vi "New File&Save Test Info_SubVIs-某型振动实验台测试系统.vi"(6 "测试条件":T3, 7 "粉尘特性":T2, 8 "error in":errorcluster, 9 "Task Info.Accele Task":T1[](array[typedef]), 11 "Test Info":cluster{"Test Name":string, "Tester":string}) -> (0 "error out":errorcluster)   [LabVIEW 2011]
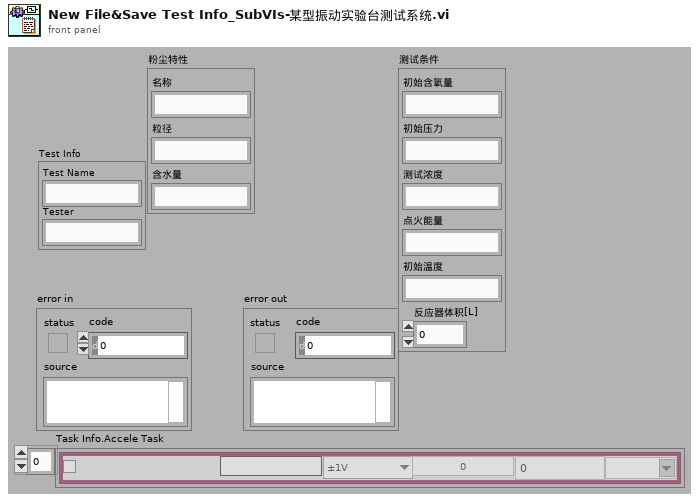
[diagram p1: front panel]
types:
  T1 = typedef "Acceleration Channel Config_Ctrls-某型振动实验台测试系统.ctl" = cluster{"Enable":bool, "Name":string, "range":enum16{"±1V", "±5V"}, "SensValue":dbl, "PhysicalName":string, "off":dbl, "Sensunits":string}
  T2 = typedef "粉尘特性.ctl" = cluster{"名称":string, "粒径":string, "含水量":string}
  T3 = typedef "测试条件.ctl" = cluster{"初始含氧量":string, "初始压力":string, "测试浓度":string, "点火能量":string, "初始温度":string, "反应器体积[L]":dbl}
  T4 = typedef "Enum File IO - FGV(V)_Ctrls-某型振动实验台测试系统.ctl" = enum16{"New", "Open", "Write Info", "Write Data", "Read Info", "Read Chan Names", "Read Data", "Close", "None"}
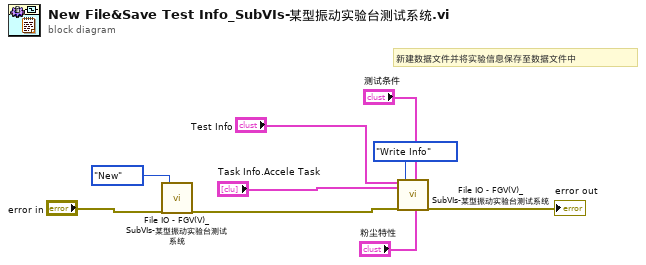
[diagram p0: block diagram]
diagram:
  # "新建数据文件并将实验信息保存至数据文件中"
  n1 = call "File IO - FGV(V)_SubVIs-某型振动实验台测试系统.vi"("error in"="error in", "Operation"=Enum_File_IO_-_FGV(V)_Ctrls-某型振动实验台测试系统."New") -> ("error out"=w6:errorcluster)  [unwired: 8 in, 9 out]
  n2 = call "File IO - FGV(V)_SubVIs-某型振动实验台测试系统.vi"("Test Info"="Test Info", "Task Info.Accele Task"="Task Info.Accele Task", "error in"=w6, "Operation"=Enum_File_IO_-_FGV(V)_Ctrls-某型振动实验台测试系统."Write Info", "测试条件"="测试条件", "粉尘特性"="粉尘特性") -> ("error out"=→"error out":errorcluster)  [unwired: 4 in, 9 out]
